vi "Get IO.vi"(8 "error in (no error)":errorcluster, 11 "Item Ref in":T1 format="%.0x") -> (0 "error out":errorcluster, 2 "IO":T2 {"Signals"."Response"."Byte Order" items=["Little Endian", "Big Endian"]; "Signals"."Response"."Data Type" items=["Signed", "Unsigned", "IEEE Float"]; "Signals"."Cmd"."Byte Order" items=["Little Endian", "Big Endian"]; "Signals"."Cmd"."Data Type" items=["Signed", "Unsigned", "IEEE Float"]}, 3 "Section Ref out":T1 format="%.0x")   [LabVIEW 2015, in "Diagnostics Addon System Explorer.lvlib"]
uses:
  Diagnostics Addon System Explorer.lvlib
  <vilib>/NI Veristand/Custom Device API/Custom Device Item Ref.ctl
  Shared/Types/IO Control Parameters.ctl
  Shared/Types/Command Response Signals.ctl
  Shared/Types/Signal Parameters.ctl
  Types/FG Action.ctl
  Get Signals.vi
  Signal Parameters FG.vi
  <vilib>/NI Veristand/Custom Device API/NI VeriStand - Get Custom Device Channel Data.vi
  <vilib>/NI Veristand/Custom Device API/NI VeriStand - Get Item Property.vi
  <vilib>/NI Veristand/Custom Device API/Get Item Property (String).vi
  <vilib>/NI Veristand/Custom Device API/Get Item Property (Double).vi
  <vilib>/NI Veristand/Custom Device API/Get Item Property (U32).vi
  <vilib>/NI Veristand/Custom Device API/NI VeriStand - Set Item Property.vi
  <vilib>/NI Veristand/Custom Device API/Set Item Property (String).vi
  <vilib>/NI Veristand/Custom Device API/Set Item Property (Double).vi
  <vilib>/NI Veristand/Custom Device API/Set Item Property (U32).vi
  Shared/SubVIs/GUID Lookup.vi
  <vilib>/NI Veristand/Custom Device API/NI VeriStand - Get Item Children.vi
  <vilib>/NI Veristand/Custom Device Tools/Custom Device Utility Library/NI VeriStand - Search for Item.vi
  <vilib>/NI Veristand/Custom Device Tools/Custom Device Utility Library/NI VeriStand - Search for Item by GUID.vi
  Shared/Diagnostics Addon Shared.lvlib
  <vilib>/NI Veristand/Custom Device API/Custom Device API.lvlib
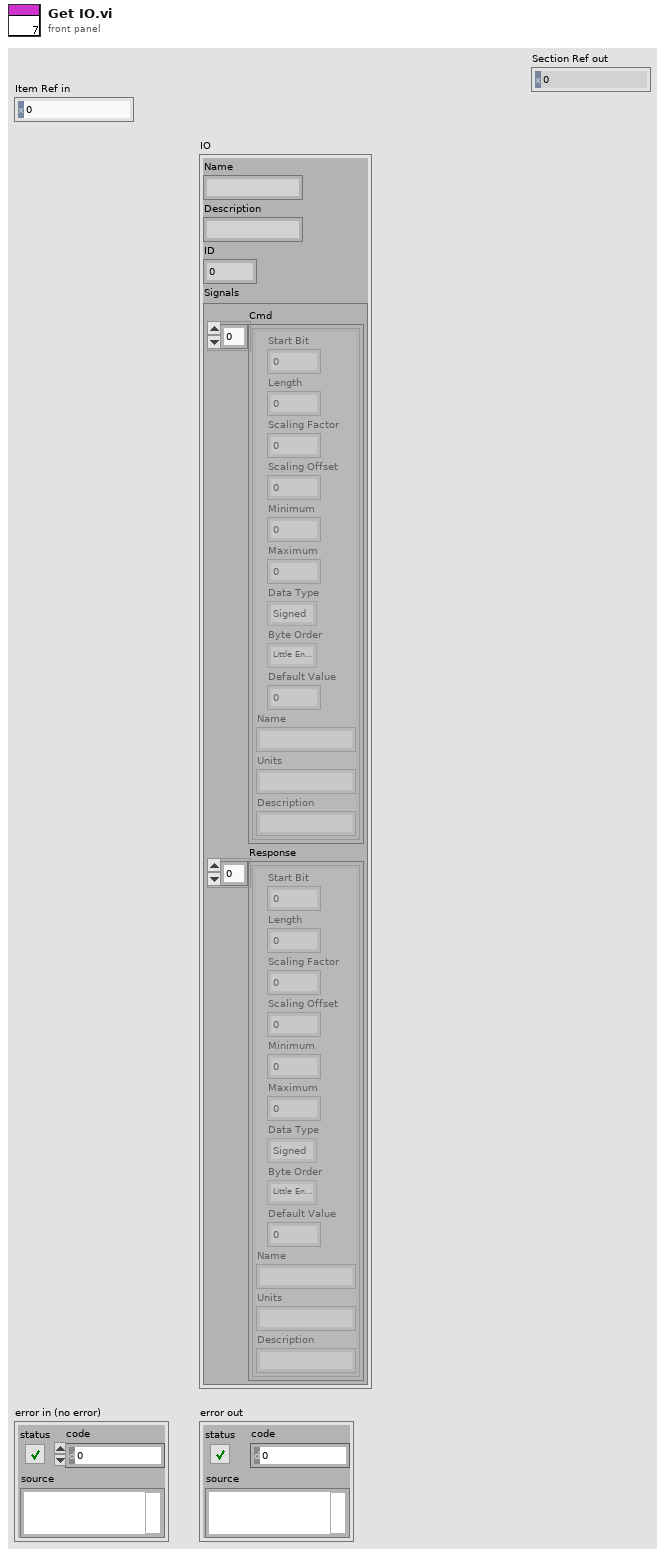
[diagram p1: front panel]
types:
  T1 = typedef "Custom Device API.lvlib/Custom Device Item Ref.ctl" = u64
  T2 = typedef "Diagnostics Addon Shared.lvlib/IO Control Parameters.ctl" = cluster{"Name":string, "Description":string, "ID":u16, "Signals":T3}
  T3 = typedef "Diagnostics Addon Shared.lvlib/Command Response Signals.ctl" = cluster{"Cmd":T4[], "Response":T4[]}
  T4 = typedef "Diagnostics Addon Shared.lvlib/Signal Parameters.ctl" = cluster{"Start Bit":u8, "Length":u8, "Scaling Factor":dbl, "Scaling Offset":dbl, "Minimum":dbl, "Maximum":dbl, "Data Type":u32, "Byte Order":u32, "Default Value":dbl, "Name":string, "Units":string, "Description":string}
  T5 = typedef "Diagnostics Addon System Explorer.lvlib/FG Action.ctl" = enum16{"Get", "Set"}
  T6 = typedef "Custom Device API.lvlib/Custom Device Item Info.ctl" = cluster{"Name":string, "Is Channel":bool, "GUID":string, "Is Waveform":bool}
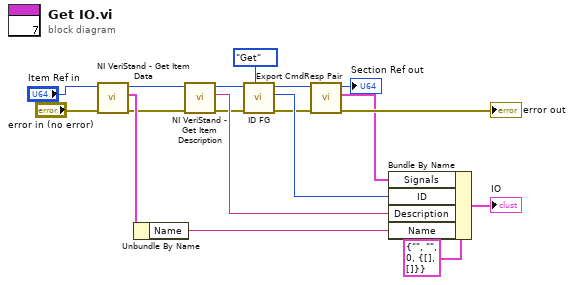
[diagram p0: block diagram]
diagram:
  n1 = call <vilib>:"NI VeriStand - Get Item Data.vi"("error in (no error)"="error in (no error)", "Item Ref in"="Item Ref in") -> ("error out"=w15:errorcluster, "Item Info"=w16:T6, "Item Ref out"=w13:T1)  [unwired: 6 in, 1 out]
  n2 = Unbundle By Name(w16) -> ("Name"=w17:string)
  n3 = call <vilib>:"NI VeriStand - Get Item Description.vi"("error in (no error)"=w15, "Item Ref in"=w13) -> ("error out"=w8:errorcluster, "Description"=w10:string, "Item Ref out"=w9:T1)  [unwired: 6 in, 1 out]
  n4 = call "ID FG.vi"("Action"=FG_Action."Get", "error in (no error)"=w8, "Device Item Ref in"=w9) -> ("error out"=w5:errorcluster, "ID"=w11:u32, "Device Item Ref out"=w4:T1)  [unwired: 6 in]
  n5 = call "Export CmdResp Pair.vi"("error in (no error)"=w5, "Device Item Ref in"=w4) -> ("error out"=→"error out":errorcluster, "Signals"=w2:T3, "Section Ref out"=→"Section Ref out":T1)  [unwired: 7 in]
  n6 = Bundle By Name(cluster=T2 {"Name"="", "Description"="", "ID"=0, "Signals"={"Cmd"=[], "Response"=[]}} ("IO"), "Signals"=w2, "ID"=w11, "Description"=w10, "Name"=w17) -> (→"IO":T2)
